vi "Set Dependent File Node.vi"(7 "type":i32(ring)=2 items=["Absolute", "Relative", "ToCommonDocDir", "ToApplicationDataDir"], 8 "error in (no error)":errorcluster, 9 "Dependent File info":T1, 10 "Property name":string, 11 ".NET Refnum in":refnum<k24>) -> (0 "error out":errorcluster, 2 "SetDependentFileValue":bool, 3 ".NET Refnum out":refnum<k24>)   [LabVIEW 2019, in "TemplatePPL System Explorer.lvlib"]
uses:
  TemplatePPL System Explorer.lvlib
  NationalInstruments.VeriStand.SystemStorage
  <vilib>/NI/NI VeriStand Advanced SysDef API/_Types/Property.DependentFile.ctl
  <vilib>/NI/NI VeriStand Advanced SysDef API/SysDef API/Advanced System Definition.lvlib
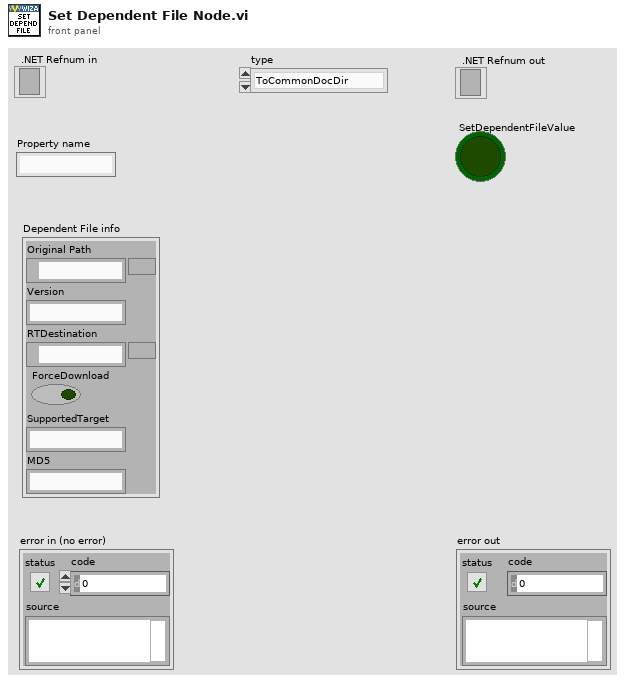
[diagram p1: front panel]
types:
  T1 = typedef "Advanced System Definition.lvlib/Property.DependentFile.ctl" = cluster{"Original Path":path, "Version":string, "RTDestination":path, "ForceDownload":bool, "SupportedTarget":string, "MD5":string}
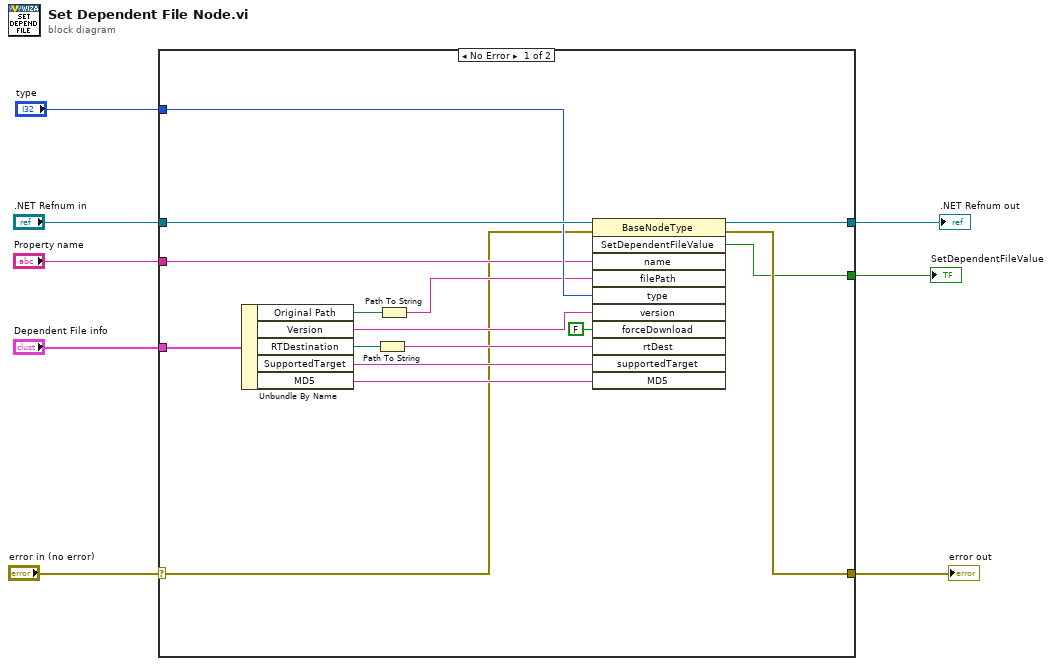
[diagram p0: block diagram]
diagram:
  n1 = case shown="No Error" "error in (no error)" {
    selector: "error in (no error)" -> [w9 w25]
    tunnel: ".NET Refnum in" -> [w24 w26]
    tunnel: [w23 w25] -> w7
    tunnel: "type" -> [w21 _]
    tunnel: "Dependent File info" -> [w20 _]
    tunnel: "Property name" -> [w12 _]
    tunnel: [w11 w26] -> w3
    tunnel: [w10 _] -> w2
    frame No Error {
      n2 = Unbundle By Name(w20) -> ("Original Path"=w19:path, "Version"=w17:string, "RTDestination"=w16:path, "SupportedTarget"=w14:string, "MD5"=w13:string)
      n3 = Path To String(path=w16) -> (string=w15:string)
      n4 = Path To String(path=w19) -> (string=w18:string)
      n5 = invoke class="BaseNodeType" method="SetDependentFileValue"(reference=w24, error in=w9, "name"=w12, "filePath"=w18, "type"=w21, "version"=w17, "forceDownload"=FALSE, "rtDest"=w15, "supportedTarget"=w14, "MD5"=w13) -> (reference out=w11:refnum<k24>, error out=w23:errorcluster, "SetDependentFileValue"=w10:bool)  [unwired: 1 in, 8 out]
    }
    frame Error {
    }
  }
  "error out" <- w7
  ".NET Refnum out" <- w3
  "SetDependentFileValue" <- w2
